vi "lab1_queue.vi"() -> ()   [LabVIEW 2014]
uses:
  sub_var_stop.vi
panel:
  in  "Array":i32[](array[numeric])=[1, 1, 1, 2, 2, 2]
  out "element":i32[](array[numeric])
  in  "Boolean":bool
  in  "stop":bool
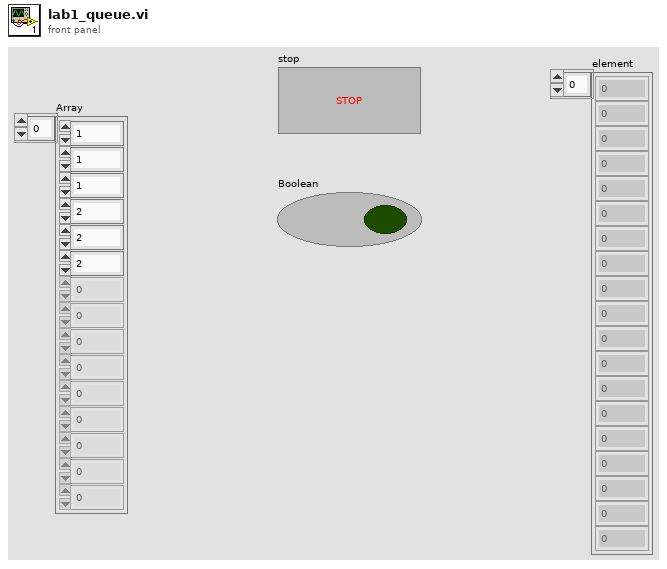
[diagram p1: front panel]
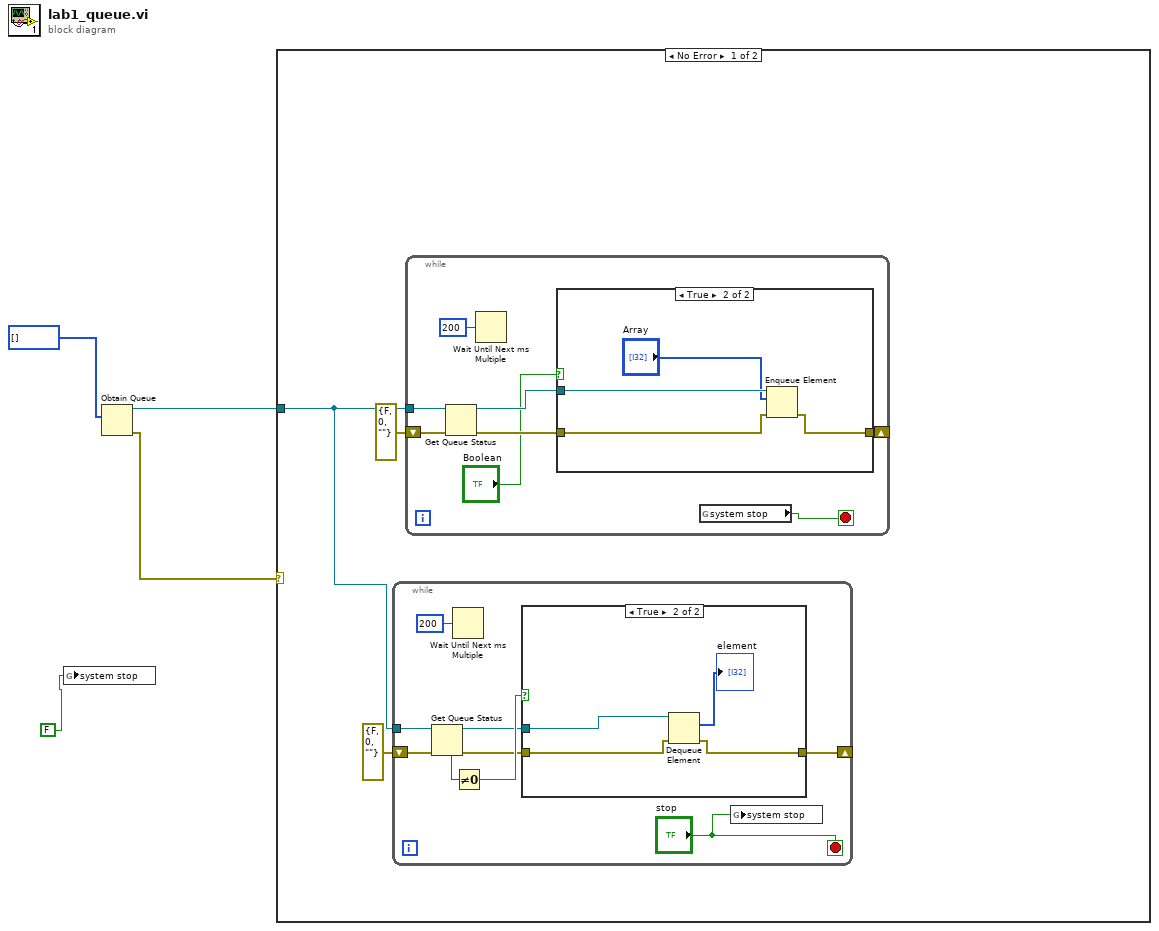
[diagram p0: block diagram]
diagram:
  n1 = global write "sub_var_stop.vi" "system stop"(FALSE) -> ()
  n2 = Obtain Queue(element data type=i32[] []) -> (queue out=w3:refnum<queue>, error out=w2:errorcluster)  [unwired: 4 in, 1 out]
  n3 = case shown="No Error" w2 {
    tunnel: w3 -> [w5 _]
    frame No Error {
      n4 = while {
        tunnel: w5 -> [w15]
        shift-right: [w9] -> _
        shift-left: errorcluster {"status"=FALSE, "code"=0, "source"=""} ("error out") -> [w10]
        stop <- "stop" stop-if-true
        n5 = Get Queue Status(queue=w15, error in (no error)=w10) -> (queue out=w12:refnum<queue>, error out=w11:errorcluster, # elements in queue=w14:i32)  [unwired: 1 in, 5 out]
        n6 = Wait Until Next ms Multiple(millisecond multiple=u32 200) -> ()  [unwired: 1 out]
        n7 = Not Equal To 0?(x=w14) -> (x != 0?=w13:bool)
        n8 = case shown="True" w13 {
          tunnel: w12 -> [_ w21]
          tunnel: w11 -> [w17 w20]
          tunnel: [w17 w19] -> w9
          frame False {
          }
          frame True {
            n9 = Dequeue Element(queue=w21, error in (no error)=w20) -> (element=→"element":i32[], error out=w19:errorcluster)  [unwired: 1 in, 2 out]
          }
        }
        n10 = global write "sub_var_stop.vi" "system stop"("stop") -> ()
      }
      n11 = while {
        tunnel: w5 -> [w29]
        shift-right: [w25] -> _
        shift-left: errorcluster {"status"=FALSE, "code"=0, "source"=""} ("error out") -> [w28]
        stop <- w22 stop-if-true
        n12 = Get Queue Status(queue=w29, error in (no error)=w28) -> (queue out=w26:refnum<queue>, error out=w24:errorcluster)  [unwired: 1 in, 6 out]
        n13 = Wait Until Next ms Multiple(millisecond multiple=u32 200) -> ()  [unwired: 1 out]
        n14 = case shown="True" "Boolean" {
          tunnel: w26 -> [_ w34]
          tunnel: [w30 w33] -> w25
          tunnel: w24 -> [w30 w32]
          frame False {
          }
          frame True {
            n15 = Enqueue Element(queue=w34, element="Array", error in (no error)=w32) -> (error out=w33:errorcluster)  [unwired: 1 in, 2 out]
          }
        }
        n16 = global read "sub_var_stop.vi" "system stop"() -> (w22:bool)
      }
    }
    frame Error {
    }
  }
